vi "Set DBL Array.vi"(7 "Treatment of Infinity/NaN":T1, 8 "error in (no error)":errorcluster, 10 "Array of numbers":dbl[](array[numeric]), 11 "JSON Array in":refnum<class "JSON Array.lvclass">) -> (0 "error out":errorcluster, 3 "JSON Array out":refnum<class "JSON Array.lvclass">)   [LabVIEW 2011, in "JSON Array.lvclass"]
uses:
  JSON Array.lvclass
  JSON Scalar/Infinity&NaN.ctl
  JSON Array.lvclass/JSON Array.ctl
  JSON Scalar/JSON Scalar.lvclass
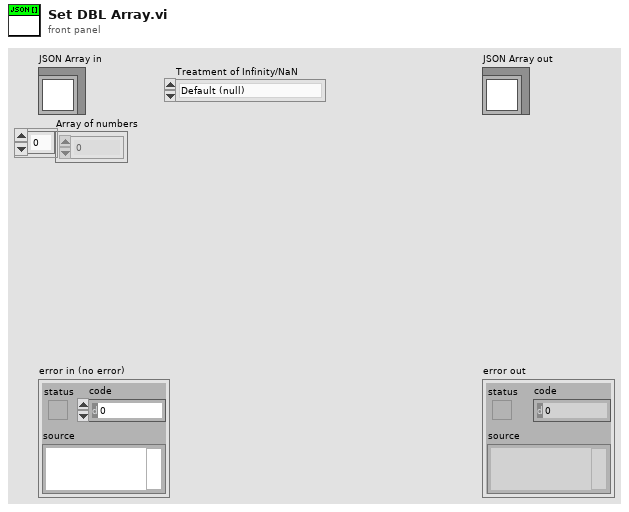
[diagram p1: front panel]
types:
  T1 = typedef "JSON Scalar.lvclass/Infinity&NaN.ctl" = enum16{"Default (null)", "Extended", "LabVIEW extensions"}
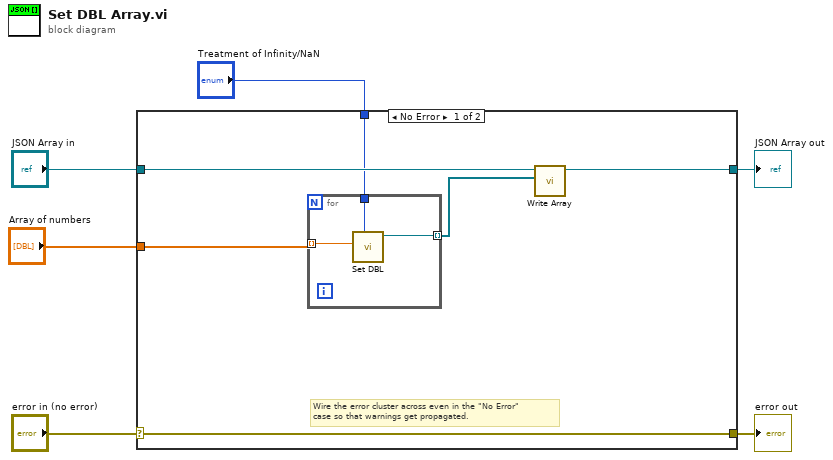
[diagram p0: block diagram]
diagram:
  n1 = case shown="No Error" "error in (no error)" {
    selector: "error in (no error)" -> [w12 w17]
    tunnel: [w12 w17] -> w5
    tunnel: [w10 w16] -> w3
    tunnel: "JSON Array in" -> [w9 w16]
    tunnel: "Array of numbers" -> [w11 _]
    tunnel: "Treatment of Infinity/NaN" -> [w7 _]
    frame No Error {
      # "Wire the error cluster across even in the \"No Error\"\ncase so that warnings get propagated."
      n2 = for {
        tunnel: w11 -> [w15] mode=indexing
        tunnel: [w14] -> w8 mode=indexing
        tunnel: w7 -> [w13]
        n3 = call "Set DBL.vi"("Treatment of Infinity/NaN"=w13, "Numeric"=w15) -> ("JSON Scalar out"=w14:refnum<class "JSON Scalar.lvclass">)  [unwired: 8 in, 1 out]
      }
      n4 = call "Write Array.vi"("Array"=w8, "JSON Array in"=w9) -> ("JSON Array out"=w10:refnum<class "JSON Array.lvclass">)  [unwired: 8 in, 1 out]
    }
    frame Error {
    }
  }
  "error out" <- w5
  "JSON Array out" <- w3
